vi "PH_DeformableMirror.ProcCases.vi"(0 "i ref in":refnum<vi>, 1 "selector":string, 2 "Data":T1, 3 "call cluster":T2={"Object"="", "Selector"="", "CallType"=enum."synchronous", "Async Object"="", "Async Selector"="", "Data Descriptor"="", "Data"=[], "Error #"=0, "Expire"=0}, 5 "error in (no error)":errorcluster) -> (14 "i ref out":refnum<vi>, 17 "answer cluster":T2={"Object"="", "Selector"="", "CallType"=enum."synchronous", "Async Object"="", "Async Selector"="", "Data Descriptor"="", "Data"=[], "Error #"=0, "Expire"=0}, 19 "error out":errorcluster)   [LabVIEW 2014, in "PH_DeformableMirror.lvlib"]
doc: "This method is called by a process from within the default case in the event loop. The methods of a class that are linked to events will be called from THIS method. Add your code here."
uses:
  PH_DeformableMirror.lvlib
  CSCore/CSSystem/CoreDefs/CoreDefs.call_type.ctl
  CSCore/BaseProcess/BaseProcess.descriptor string definition.ctl
  CSCore/CSSystem/CoreDefs/CoreDefs.rawDataType.ctl
  CSCore/CSSystem/CoreLib/CoreLib.byte array 2 short.vi
  CSCore/CSSystem/CoreLib/CoreLib.string 2 byte array.vi
  CSCore/CSSystem/CoreLib/CoreLib.byte array 2 int.vi
  CSCore/CSSystem/CoreLib/CoreLib.byte array 2 double.vi
  CSCore/CSSystem/CoreLib/CoreLib.byte array 2 double array.vi
  CSCore/BaseProcess/BaseProcess.lvlib
  CSCore/CSSystem/CoreLib/CoreLib.lvlib
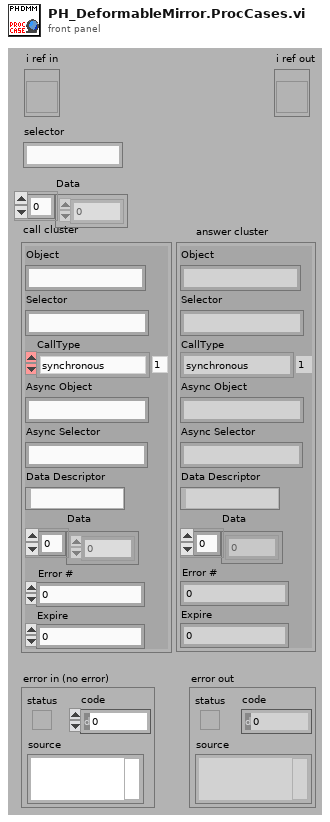
[diagram p1: front panel]
types:
  T1 = typedef "CoreDefs.rawDataType.ctl" = i8[]
  T2 = typedef "CoreDefs.call_type.ctl" = cluster{"Object":string, "Selector":string, "CallType":enum16{"simple", "synchronous", "asynchronous"}, "Async Object":string, "Async Selector":string, "Data Descriptor":T3, "Data":T1, "Error #":i32, "Expire":u32}
  T3 = typedef "BaseProcess.lvlib/BaseProcess.descriptor string definition.ctl" = string
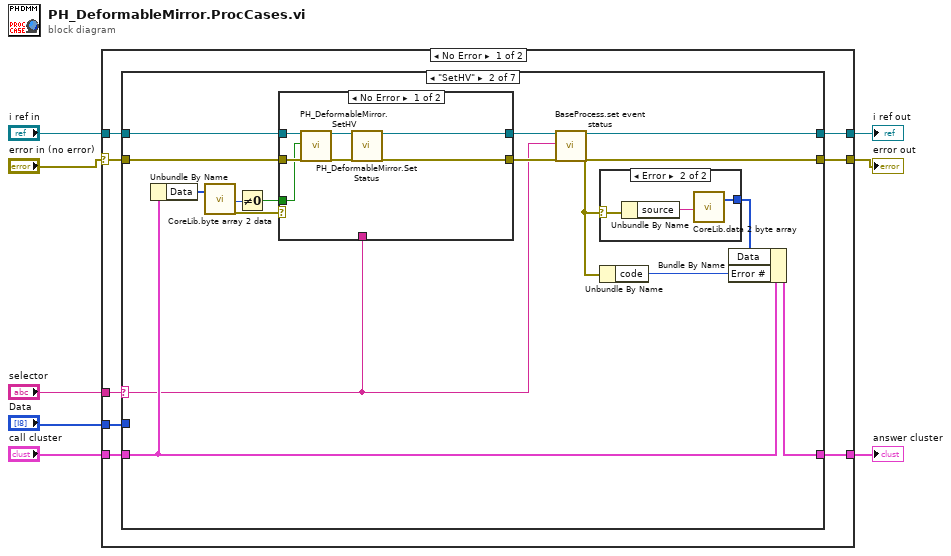
[diagram p0: block diagram]
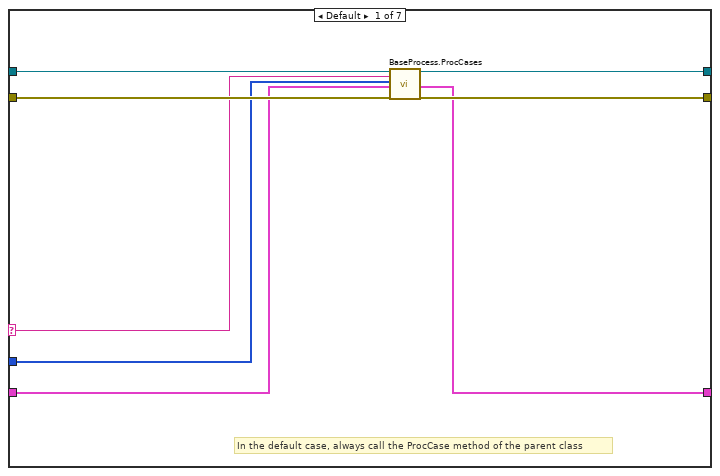
[diagram p2: hidden frame]
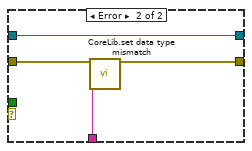
[diagram p4: hidden frame]
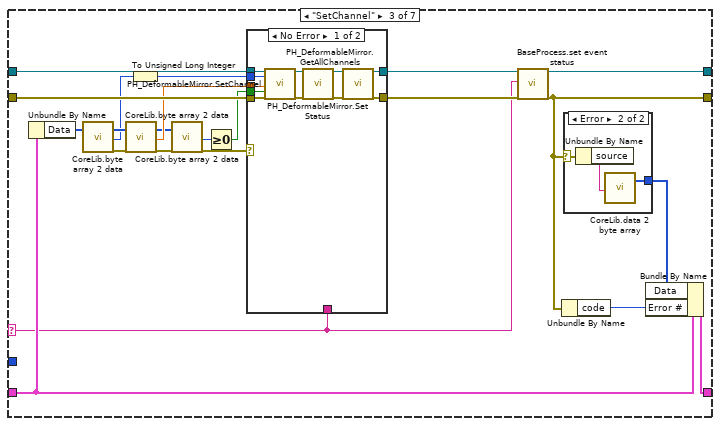
[diagram p5: hidden frame]
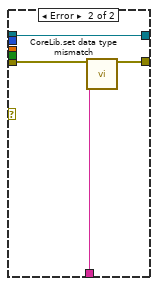
[diagram p7: hidden frame]
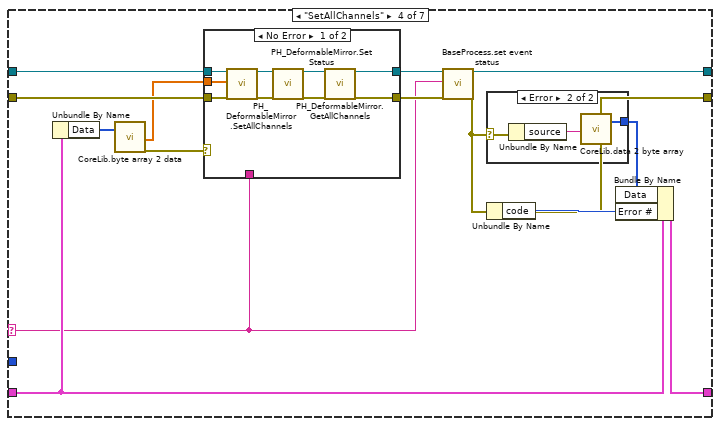
[diagram p8: hidden frame]
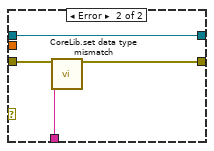
[diagram p10: hidden frame]
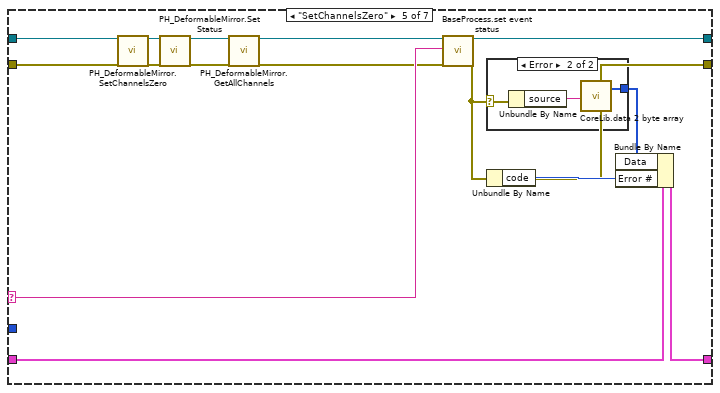
[diagram p11: hidden frame]
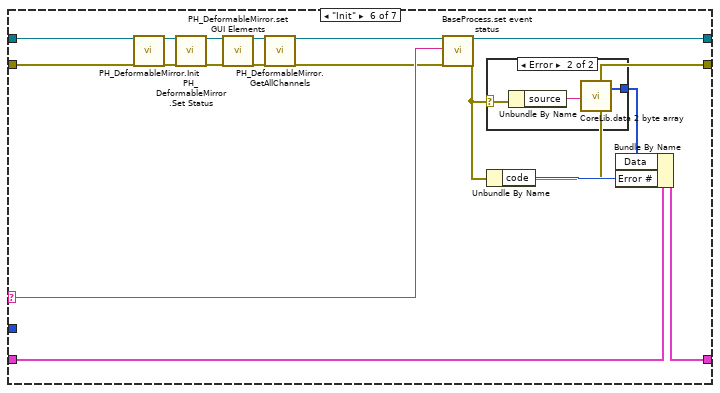
[diagram p13: hidden frame]
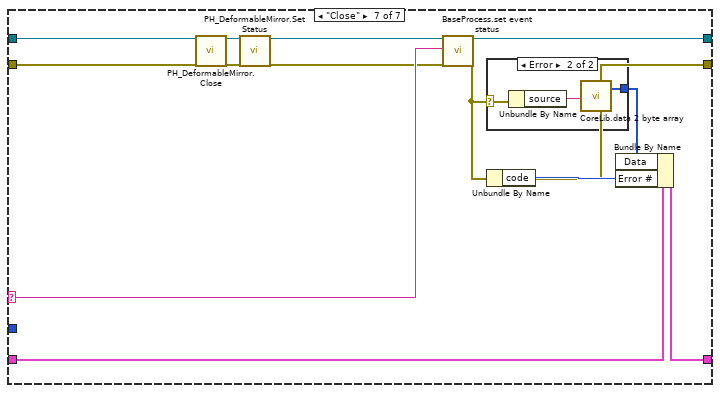
[diagram p15: hidden frame]
diagram:
  n1 = case shown="No Error" "error in (no error)" {
    selector: "error in (no error)" -> [w9 w178]
    tunnel: "selector" -> [w16 _]
    tunnel: [w15 w179] -> w7
    tunnel: "Data" -> [w14 _]
    tunnel: "call cluster" -> [w13 w179]
    tunnel: "i ref in" -> [w12 w180]
    tunnel: [w11 w180] -> w3
    tunnel: [w10 w178] -> w2
    frame No Error {
      n2 = case shown="\"SetHV\"" w16 {
        selector: w16 -> [w18 w30 w66 w98 w131 w151 w167]
        tunnel: w14 -> [w19 _ _ _ _ _ _]
        tunnel: w12 -> [w17 w39 w75 w107 w138 w158 w174]
        tunnel: [w24 w29 w65 w97 w130 w150 w166] -> w11
        tunnel: w13 -> [w20 w36 w72 w104 w135 w155 w171]
        tunnel: [w21 w35 w71 w103 w134 w154 w170] -> w15
        tunnel: w9 -> [w23 w38 w74 w106 w137 w157 w173]
        tunnel: [w22 w31 w67 w99 w132 w152 w168] -> w10
        frame Default {
          # "In the default case, always call the ProcCase method of the parent class"
          n3 = call "BaseProcess.ProcCases.vi"("i ref in"=w17, "selector"=w18, "Data"=w19, "call cluster"=w20, "error in (no error)"=w23) -> ("i ref out"=w24:refnum<vi>, "answer cluster"=w21:T2, "error out"=w22:errorcluster)  [unwired: 12 in]
        }
        frame "SetHV" {
          n4 = Unbundle By Name(w36) -> ("Data"=w28:T1)
          n5 = call-poly "CoreLib.byte array 2 data.vi"("byteArray"=w28) -> ("i16"=w26:i16, "error out"=w27:errorcluster)  [unwired: 16 in, 1 out]
          n6 = Not Equal To 0?(x=w26) -> (x != 0?=w25:bool)
          n7 = case shown="No Error" w27 {
            tunnel: [w43 w53] -> w33
            tunnel: w39 -> [w49 w53]
            tunnel: w38 -> [w48 w52]
            tunnel: [w45 w51] -> w32
            tunnel: w30 -> [_ w50]
            tunnel: w25 -> [w46 _]
            frame No Error {
              n8 = call "PH_DeformableMirror.SetHV.vi"("i ref in"=w49, "HV on/off"=w46, "error in"=w48) -> ("i ref out"=w44:refnum<vi>, "error out"=w47:errorcluster)  [unwired: 15 in]
              n9 = call "PH_DeformableMirror.Set Status.vi"("i ref in"=w44, "error in"=w47) -> ("i ref out"=w43:refnum<vi>, "error out"=w45:errorcluster)  [unwired: 16 in]
            }
            frame Error {
              n10 = call "CoreLib.set data type mismatch.vi"("error in (no error)"=w52, "error source"=w50) -> ("error out"=w51:errorcluster)  [unwired: 17 in]
            }
          }
          n11 = call "BaseProcess.set event status.vi"("i ref in"=w33, "EventStatus"=w30, "error in (no error)"=w32) -> ("i ref out"=w29:refnum<vi>, "error out"=w31:errorcluster)  [unwired: 14 in, 1 out]
          n12 = case shown="Error" w31 {
            selector: w31 -> [_ w42]
            tunnel: [_ w41] -> w34
            frame No Error {
            }
            frame Error {
              n13 = Unbundle By Name(w42) -> ("source"=w40:string)
              n14 = call-poly "CoreLib.data 2 byte array.vi"("string"=w40) -> ("byteArray out"=w41:T1)  [unwired: 18 in]
            }
          }
          n15 = Unbundle By Name(w31) -> ("code"=w37:i32)
          n16 = Bundle By Name(cluster=w36, "Data"=w34, "Error #"=w37) -> (w35:T2)
        }
        frame "SetChannel" {
          n17 = Unbundle By Name(w72) -> ("Data"=w64:T1)
          n18 = call-poly "CoreLib.byte array 2 data.vi"("byteArray"=w64) -> ("byteArray out"=w63:T1, "i32"=w60:i32, "error out"=w62:errorcluster)  [unwired: 16 in]
          n19 = call-poly "CoreLib.byte array 2 data.vi"("byteArray"=w63, "error in (no error)"=w62) -> ("byteArray out"=w56:T1, "d64"=w61:dbl, "error out"=w58:errorcluster)  [unwired: 15 in]
          n20 = To Unsigned Long Integer(number=w60) -> (unsigned 32bit integer=w59:u32)
          n21 = call-poly "CoreLib.byte array 2 data.vi"("byteArray"=w56, "error in (no error)"=w58) -> ("i16"=w55:i16, "error out"=w57:errorcluster)  [unwired: 15 in, 1 out]
          n22 = Greater Or Equal To 0?(x=w55) -> (x >= 0?=w54:bool)
          n23 = case shown="No Error" w57 {
            tunnel: [w81 w93] -> w69
            tunnel: w75 -> [w89 w93]
            tunnel: w74 -> [w88 w92]
            tunnel: [w80 w91] -> w68
            tunnel: w66 -> [_ w90]
            tunnel: w61 -> [w86 _]
            tunnel: w59 -> [w87 _]
            tunnel: w54 -> [w79 _]
            frame No Error {
              n24 = call "PH_DeformableMirror.SetChannel.vi"("i ref in"=w89, "Channel"=w87, "Voltage"=w86, "Hysteresis Compensation? (false)"=w79, "error in"=w88) -> ("i ref out"=w85:refnum<vi>, "error out"=w84:errorcluster)  [unwired: 13 in]
              n25 = call "PH_DeformableMirror.Set Status.vi"("i ref in"=w85, "error in"=w84) -> ("i ref out"=w82:refnum<vi>, "error out"=w83:errorcluster)  [unwired: 16 in]
              n26 = call "PH_DeformableMirror.GetAllChannels.vi"("VI in"=w82, "error in (no error)"=w83) -> ("VI out"=w81:refnum<vi>, "error out"=w80:errorcluster)  [unwired: 16 in]
            }
            frame Error {
              n27 = call "CoreLib.set data type mismatch.vi"("error in (no error)"=w92, "error source"=w90) -> ("error out"=w91:errorcluster)  [unwired: 17 in]
            }
          }
          n28 = call "BaseProcess.set event status.vi"("i ref in"=w69, "EventStatus"=w66, "error in (no error)"=w68) -> ("i ref out"=w65:refnum<vi>, "error out"=w67:errorcluster)  [unwired: 14 in, 1 out]
          n29 = Unbundle By Name(w67) -> ("code"=w73:i32)
          n30 = case shown="Error" w67 {
            selector: w67 -> [_ w78]
            tunnel: [_ w77] -> w70
            frame No Error {
            }
            frame Error {
              n31 = Unbundle By Name(w78) -> ("source"=w76:string)
              n32 = call-poly "CoreLib.data 2 byte array.vi"("string"=w76) -> ("byteArray out"=w77:T1)  [unwired: 18 in]
            }
          }
          n33 = Bundle By Name(cluster=w72, "Data"=w70, "Error #"=w73) -> (w71:T2)
        }
        frame "SetAllChannels" {
          n34 = Unbundle By Name(w104) -> ("Data"=w96:T1)
          n35 = call-poly "CoreLib.byte array 2 data.vi"("byteArray"=w96) -> ("[d64]"=w95:dbl[], "error out"=w94:errorcluster)  [unwired: 16 in, 1 out]
          n36 = case shown="No Error" w94 {
            tunnel: [w113 w123] -> w101
            tunnel: w107 -> [w118 w123]
            tunnel: w106 -> [w117 w122]
            tunnel: [w111 w121] -> w100
            tunnel: w98 -> [_ w120]
            tunnel: w95 -> [w119 _]
            frame No Error {
              n37 = call "PH_DeformableMirror.SetAllChannels.vi"("i ref in"=w118, "Voltages"=w119, "error in"=w117) -> ("i ref out"=w116:refnum<vi>, "error out"=w115:errorcluster)  [unwired: 15 in]
              n38 = call "PH_DeformableMirror.Set Status.vi"("i ref in"=w116, "error in"=w115) -> ("i ref out"=w114:refnum<vi>, "error out"=w112:errorcluster)  [unwired: 16 in]
              n39 = call "PH_DeformableMirror.GetAllChannels.vi"("VI in"=w114, "error in (no error)"=w112) -> ("VI out"=w113:refnum<vi>, "error out"=w111:errorcluster)  [unwired: 16 in]
            }
            frame Error {
              n40 = call "CoreLib.set data type mismatch.vi"("error in (no error)"=w122, "error source"=w120) -> ("error out"=w121:errorcluster)  [unwired: 17 in]
            }
          }
          n41 = call "BaseProcess.set event status.vi"("i ref in"=w101, "EventStatus"=w98, "error in (no error)"=w100) -> ("i ref out"=w97:refnum<vi>, "error out"=w99:errorcluster)  [unwired: 14 in, 1 out]
          n42 = case shown="Error" w99 {
            selector: w99 -> [_ w110]
            tunnel: [_ w109] -> w102
            frame No Error {
            }
            frame Error {
              n43 = Unbundle By Name(w110) -> ("source"=w108:string)
              n44 = call-poly "CoreLib.data 2 byte array.vi"("string"=w108) -> ("byteArray out"=w109:T1)  [unwired: 18 in]
            }
          }
          n45 = Unbundle By Name(w99) -> ("code"=w105:i32)
          n46 = Bundle By Name(cluster=w104, "Data"=w102, "Error #"=w105) -> (w103:T2)
        }
        frame "SetChannelsZero" {
          n47 = call "PH_DeformableMirror.SetChannelsZero.vi"("i ref in"=w138, "error in"=w137) -> ("i ref out"=w129:refnum<vi>, "error out"=w128:errorcluster)  [unwired: 16 in]
          n48 = call "PH_DeformableMirror.Set Status.vi"("i ref in"=w129, "error in"=w128) -> ("i ref out"=w127:refnum<vi>, "error out"=w125:errorcluster)  [unwired: 16 in]
          n49 = call "PH_DeformableMirror.GetAllChannels.vi"("VI in"=w127, "error in (no error)"=w125) -> ("VI out"=w126:refnum<vi>, "error out"=w124:errorcluster)  [unwired: 16 in]
          n50 = call "BaseProcess.set event status.vi"("i ref in"=w126, "EventStatus"=w131, "error in (no error)"=w124) -> ("i ref out"=w130:refnum<vi>, "error out"=w132:errorcluster)  [unwired: 14 in, 1 out]
          n51 = case shown="Error" w132 {
            selector: w132 -> [_ w141]
            tunnel: [_ w140] -> w133
            frame No Error {
            }
            frame Error {
              n52 = Unbundle By Name(w141) -> ("source"=w139:string)
              n53 = call-poly "CoreLib.data 2 byte array.vi"("string"=w139) -> ("byteArray out"=w140:T1)  [unwired: 18 in]
            }
          }
          n54 = Unbundle By Name(w132) -> ("code"=w136:i32)
          n55 = Bundle By Name(cluster=w135, "Data"=w133, "Error #"=w136) -> (w134:T2)
        }
        frame "Init" {
          n56 = call "PH_DeformableMirror.Init.vi"("VI in"=w158, "error in (no error)"=w157) -> ("VI out"=w148:refnum<vi>, "error out"=w149:errorcluster)  [unwired: 16 in]
          n57 = call "PH_DeformableMirror.Set Status.vi"("i ref in"=w148, "error in"=w149) -> ("i ref out"=w147:refnum<vi>, "error out"=w146:errorcluster)  [unwired: 16 in]
          n58 = call "PH_DeformableMirror.set GUI Elements.vi"("VI in"=w147, "error in (no error)"=w146) -> ("VI out"=w145:refnum<vi>, "error out"=w143:errorcluster)  [unwired: 16 in]
          n59 = call "PH_DeformableMirror.GetAllChannels.vi"("VI in"=w145, "error in (no error)"=w143) -> ("VI out"=w144:refnum<vi>, "error out"=w142:errorcluster)  [unwired: 16 in]
          n60 = call "BaseProcess.set event status.vi"("i ref in"=w144, "EventStatus"=w151, "error in (no error)"=w142) -> ("i ref out"=w150:refnum<vi>, "error out"=w152:errorcluster)  [unwired: 14 in, 1 out]
          n61 = case shown="Error" w152 {
            selector: w152 -> [_ w161]
            tunnel: [_ w160] -> w153
            frame No Error {
            }
            frame Error {
              n62 = Unbundle By Name(w161) -> ("source"=w159:string)
              n63 = call-poly "CoreLib.data 2 byte array.vi"("string"=w159) -> ("byteArray out"=w160:T1)  [unwired: 18 in]
            }
          }
          n64 = Unbundle By Name(w152) -> ("code"=w156:i32)
          n65 = Bundle By Name(cluster=w155, "Data"=w153, "Error #"=w156) -> (w154:T2)
        }
        frame "Close" {
          n66 = call "PH_DeformableMirror.Close.vi"("VI in"=w174, "error in (no error)"=w173) -> ("VI out"=w163:refnum<vi>, "error out"=w162:errorcluster)  [unwired: 16 in]
          n67 = call "PH_DeformableMirror.Set Status.vi"("i ref in"=w163, "error in"=w162) -> ("i ref out"=w165:refnum<vi>, "error out"=w164:errorcluster)  [unwired: 16 in]
          n68 = call "BaseProcess.set event status.vi"("i ref in"=w165, "EventStatus"=w167, "error in (no error)"=w164) -> ("i ref out"=w166:refnum<vi>, "error out"=w168:errorcluster)  [unwired: 14 in, 1 out]
          n69 = case shown="Error" w168 {
            selector: w168 -> [_ w177]
            tunnel: [_ w176] -> w169
            frame No Error {
            }
            frame Error {
              n70 = Unbundle By Name(w177) -> ("source"=w175:string)
              n71 = call-poly "CoreLib.data 2 byte array.vi"("string"=w175) -> ("byteArray out"=w176:T1)  [unwired: 18 in]
            }
          }
          n72 = Unbundle By Name(w168) -> ("code"=w172:i32)
          n73 = Bundle By Name(cluster=w171, "Data"=w169, "Error #"=w172) -> (w170:T2)
        }
      }
    }
    frame Error {
    }
  }
  "answer cluster" <- w7
  "i ref out" <- w3
  "error out" <- w2
